vi "Thermometer SUB.vi"(0 "Slide":dbl, 1 "Boolean":bool) -> (14 "Numeric":dbl)   [LabVIEW 2023]
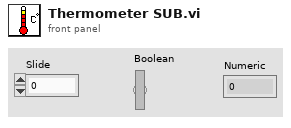
[diagram p1: front panel]
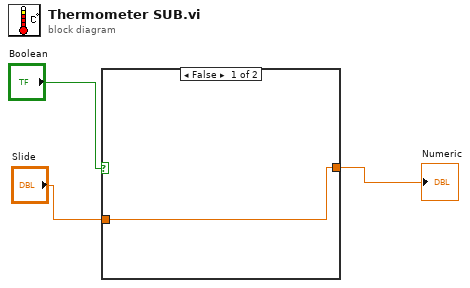
[diagram p0: block diagram]
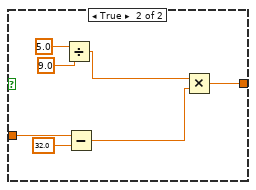
[diagram p2: hidden frame]
diagram:
  n1 = case shown="False" "Boolean" {
    tunnel: [w4 w7] -> w3
    tunnel: "Slide" -> [w4 w5]
    frame False {
    }
    frame True {
      n2 = Divide(x=5.0, y=9.0) -> (x/y=w9:dbl)
      n3 = Subtract(x=w5, y=32.0) -> (x-y=w8:dbl)
      n4 = Multiply(x=w9, y=w8) -> (x*y=w7:dbl)
    }
  }
  "Numeric" <- w3
